vi "ChangeFileExtention.vi"(8 "File Extension Separator (.)":string=".", 10 "New Extention":string, 11 "Path":path) -> (0 "Name with new extension":string, 1 "Path with new extension":path, 2 "Name before extension":string, 3 "Path before extension":path, 4 "Old Extension":string)   [LabVIEW 2015]
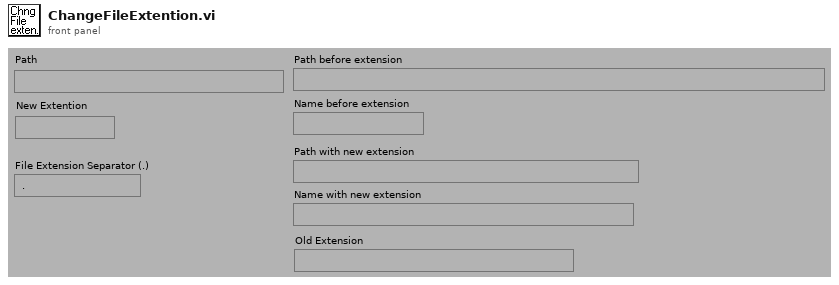
[diagram p1: front panel]
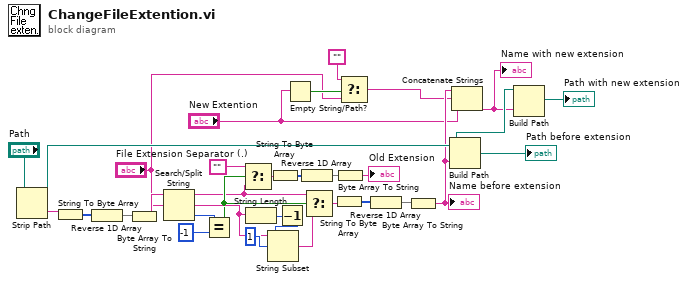
[diagram p0: block diagram]
diagram:
  n1 = Strip Path(path="Path") -> (stripped path=w17:path, name=w31:string)
  n2 = String To Byte Array(string=w31) -> (unsigned byte array=w30:u8[])
  n3 = Reverse 1D Array(array=w30) -> (reversed array=w29:u8[])
  n4 = Byte Array To String(unsigned byte array=w29) -> (string=w28:string)
  n5 = Search/Split String(string=w28, search string/char (-)="File Extension Separator (.)") -> (substring before match=w14:string, match + rest of string=w23:string, offset of match=w27:i32)  [unwired: 1 out]
  n6 = Equal?(x=w27, y=-1) -> (x = y?=w15:bool)
  n7 = Select(t="", s=w15, f=w14) -> (s? t:f=w11:string)
  n8 = String Length(string=w23) -> (length=w21:i32)
  n9 = String To Byte Array(string=w11) -> (unsigned byte array=w13:u8[])
  n10 = Decrement(x=w21) -> (x-1=w22:i32)
  n11 = String Subset(string=w23, offset (0)=1, length (rest)=w22) -> (substring=w24:string)
  n12 = Empty String/Path?(string/path="New Extention") -> (empty?=w6:bool)
  n13 = Reverse 1D Array(array=w13) -> (reversed array=w12:u8[])
  n14 = Select(t=w14, s=w15, f=w24) -> (s? t:f=w18:string)
  n15 = String To Byte Array(string=w18) -> (unsigned byte array=w20:u8[])
  n16 = Byte Array To String(unsigned byte array=w12) -> (string=→"Old Extension":string)
  n17 = Select(t="", s=w6, f="File Extension Separator (.)") -> (s? t:f=w3:string)
  n18 = Reverse 1D Array(array=w20) -> (reversed array=w19:u8[])
  n19 = Byte Array To String(unsigned byte array=w19) -> (string=w8:string)
  "Name before extension" <- w8
  n20 = Build Path(base path=w17, name or relative path=w8) -> (appended path=→"Path before extension":path)
  n21 = Concatenate Strings(w8, w3, "New Extention") -> (w2:string)
  "Name with new extension" <- w2
  n22 = Build Path(base path=w17, name or relative path=w2) -> (appended path=→"Path with new extension":path)
